vi "WriteHSpeed.vi"(8 "error in":errorcluster, 9 "Reply length":i32=-1, 10 "write buffer":string, 11 "Python":T1) -> (0 "error out":errorcluster, 2 "read buffer":string, 3 "Python":T1)   [LabVIEW 2022 SP3]
uses:
  PythonCtrl.ctl
  Processors.ctl
panel:
  out "x = y?":bool
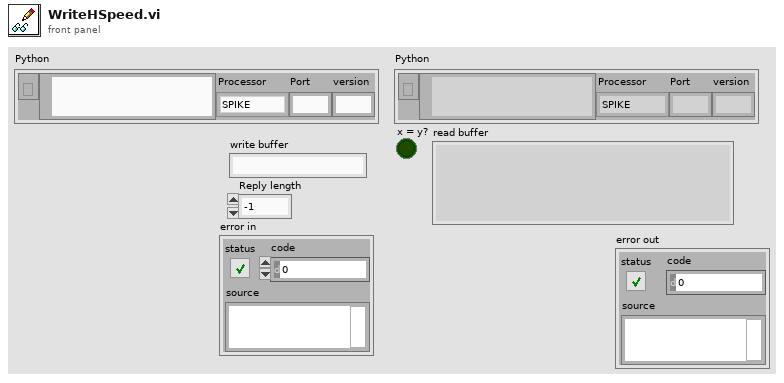
[diagram p1: front panel]
types:
  T1 = typedef "PythonCtrl.ctl" = cluster{"session":refnum<k35>, "PyPath":path, "Processor":T2, "Port":string, "version":string}
  T2 = typedef "Processors.ctl" = enum16{"SPIKE", "Pi", "Pi_ssh", "OpenMV", "Dunio"}
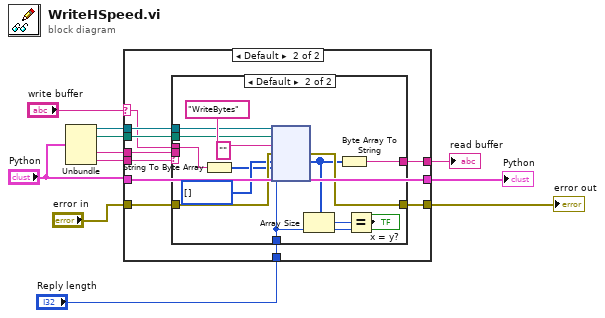
[diagram p0: block diagram]
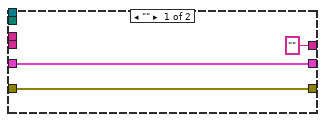
[diagram p2: hidden frame]
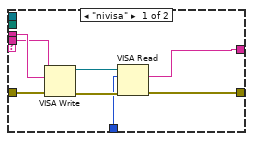
[diagram p3: hidden frame]
diagram:
  n1 = Unbundle("Python") -> ("session"=w5:refnum<k35>, "PyPath"=w4:path, "Port"=w1:string, "version"=w3:string)  [unwired: 1 out]
  n2 = case shown="Default" "write buffer" {
    selector: "write buffer" -> [_ w17]
    tunnel: "Python" -> [w14 w24]
    tunnel: "error in" -> [w13 w23]
    tunnel: [w14 w24] -> w7
    tunnel: [w13 w22] -> w6
    tunnel: "Reply length" -> [_ w21]
    tunnel: w5 -> [_ w20]
    tunnel: w4 -> [_ w19]
    tunnel: w3 -> [_ w18]
    tunnel: ["" ("string") w16] -> w2
    tunnel: w1 -> [_ w15]
    frame "" {
    }
    frame Default {
      n3 = case shown="Default" w18 {
        tunnel: w23 -> [w32 w44]
        tunnel: [w27 w43] -> w22
        tunnel: w21 -> [w29 w34]
        tunnel: w20 -> [_ w42]
        tunnel: w19 -> [_ w41]
        tunnel: w17 -> [w31 w39]
        tunnel: [w26 w37] -> w16
        tunnel: w15 -> [w25 _]
        frame "nivisa" {
          n4 = VISA Write(VISA resource name=w25, write buffer=w31, error in (no error)=w32) -> (VISA resource name out=w28:refnum<visa-resource-name>, error out=w30:errorcluster)  [unwired: 1 out]
          n5 = VISA Read(VISA resource name=w28, byte count=w29, error in (no error)=w30) -> (read buffer=w26:string, error out=w27:errorcluster)  [unwired: 2 out]
        }
        frame Default {
          (unwired) "" ("function name")
          n6 = String To Byte Array(string=w39) -> (unsigned byte array=w38:u8[])
          n7 = node(w42, w41, "WriteBytes" ("function name"), w44, u8[] [] ("unsigned byte array"), w38, w34) -> (w43:errorcluster, w36:u8[])  [unwired: 2 in, 3 out]
          n8 = Array Size(array=w36) -> (size(s)=w35:i32)
          n9 = Byte Array To String(unsigned byte array=w36) -> (string=w37:string)
          n10 = Equal?(x=w35, y=w34) -> (x = y?=→"x = y?":bool)
        }
      }
    }
  }
  "Python" <- w7
  "error out" <- w6
  "read buffer" <- w2
